vi "Initialize Session.vi"(7 "Acquisition Parameters In":T1={"Magnet Angle [deg]"=0.0, "Magnet Angles [deg]"=[], "DeltaVpp [v]"=0.0, "SEM [v]"=0.0, "DeltaVpp Thresh [v]"=0.0, "SEM Thresh [v]"=0.0, "Adaptive Processing"=FALSE, "Acquire Q"=FALSE, "Acquire Photos"=FALSE, "Adaptive Tuning"=FALSE, "Automated Matching"=FALSE, "X-Gradient [G/mm]"=0.0, "Y-Gradient [G/mm]"=0.0, "Z-Gradient [G/mm]"=0.0, "Central Field [G]"=0.0, "Scan Width [G]"=0.0, "Mod. Amp. [G]"=0.0, "Scan Time [s]"=0.0, "Pre-Scan Delay [ms]"=0, "Measurement Timeout [s]"=0.0, "Electromagnet Main Field [G]"=0.0, "Locked Central Field [G]"=0.0, "Scans Excluded"=0, "Scans Completed"=0, "No. Scans/Set"=0, "No. Scans for SNR"=0, "Field Locked Frequency [GHz]"=0.0, "Auto Set-based Field Center"=FALSE, "Prompt for oxy acquisition updates"=FALSE, "Oxy QA Scan?"=FALSE, "Exclude Bad Data"=FALSE, "Optimizing RF Power"=FALSE, "Gradients on/off"=TRUE, "Running Script"=FALSE, "Opto-Coupler Current [A]"=0.0, "Continuous Sweeping"=FALSE, "Sweep Rise Time [sec]"=0, "Reverse Sweep Central Field [G]"=0.0, "Forward Sweep Central Field [G]"=0.0, "Sweep Calibrated"=FALSE, "Modulation Calibrated"=FALSE, "First CheckCal Scan?"=FALSE, "AFC Field Correction"=FALSE, "OxyQAInit Scan Width [G]"=0.0, "OxyQAInit Mod. Amp. [G]"=0.0, "Scans Completed/Session"=0, "Acquire SpO2"=FALSE, "Acquire Temperature"=FALSE, "Over Mod"=FALSE} {"OxyQAInit Mod. Amp. [G]" min=0.0; "OxyQAInit Scan Width [G]" min=0.0; "Mod. Amp. [G]" min=0.0; "Scan Width [G]" min=0.0; "Measurement Timeout [s]" min=0.0; "Scan Time [s]" min=0.0; "Z-Gradient [G/mm]" min=0.0; "Y-Gradient [G/mm]" min=0.0; "X-Gradient [G/mm]" min=0.0; "SEM Thresh [v]" min=0.0; "DeltaVpp Thresh [v]" min=0.0; "SEM [v]" min=0.0}, 9 "Spectral Data In":T3={"PDT Amp [v]"=0.0, "RIS Amp [v]"=0.0, "B-Field"=[], "All In-Phase Scan Spectra"=[], "Model Select"=enum."OneCompRISTwoPDT", "Fit Each Scan"=FALSE, "PDT Center [g]"=0.0, "In-Phase Average Spectra"=[], "In-Phase Median Spectra"=[], "Out-Phase Median Spectra"=[], "Out-Phase Average Spectra"=[], "Fit Spectra"=[], "Fit No-Baseline Spectra"=[], "All Out-Phase Scan Spectra"=[], "Baseline Offset Correction"=FALSE, "In-Phase Offset [v]"=0.0, "Out-Phase Offset [v]"=0.0, "Ch2 Input\n(Balance)"=[], "Ch3 Input\n(Phase)"=[], "Ch4 Input\n(AFC)"=[], "Fit Pars"=[], "Fit Pars Errors"=[], "Fit Pars Labels"=[], "Raw Scan DAQ Data"=[], "Bad Scans Indicies"=[], "Good In-Phase Scan Spectra"=[], "Good Out-Phase Scan Spectra"=[], "Bad In-Phase Scan Spectra"=[], "Bad Out-Phase Scan Spectra"=[], "Number of bad scans"=0, "Fit History"=[], "PDT Amp. History/Set [v]"=[], "RIS Amp. History/Set [v]"=[], "RIS Amp. History/Scan [v]"=[], "All Shifted B-Fields"=[], "Good Shifted B-Fields"=[], "Ch5 Input\n(SpO2)"=[], "Ch6 Input\n(BPM)"=[], "Global SNR"=0.0, "Fit Error History"=[], "SNR History"=[]} {"Global SNR" min=0.0; "PDT Center [g]" min=0.0; "RIS Amp [v]" min=0.0; "PDT Amp [v]" min=0.0}, 10 "Measurement Information In":T7={"Comments"="", "Directory Input"="", "Data file path"=path "C:/Data/EPR Data", "Scripting File"=path "C:/Data/Configuration Script.csv", "Save Data"=FALSE, "Tooth size (d11) [mm]"=0.0, "Tooth size (d12) [mm]"=0.0, "Tooth size (d21) [mm]"=0.0, "Tooth size (d22) [mm]"=0.0, "Dose of Tooth [Gy]"=0.0, "Safe Shutdown?"=FALSE, "Gases Available"=[], "Database Username"="", "Database Password"="", "Database Login URL"="", "Database Upload URL"="", "Database Success URL"="", "Database XML URL"="", "Database Resonator URL"="", "Session Number"=0, "Set #"=0, "Resonator Operator"="", "Session Type"="", "Tooth/Sample ID"="", "Volunteer ID"="", "Computer Operator"="", "Volunteer Type"="", "Site/Tooth Selection (T8,T9)"="", "Resonator"="", "Measurement Site"="", "Non-standard session?"=FALSE, "EPR DAQ Version"="", "Session Path"=path "C:/Data/EPR Data", "Chosen Applied State"="", "Chosen Initial State"="", "Time of Transition"="", "DAQ Mode"=enum."Engineering", "pO2/Scan [mmHg]"=[], "pO2/Set [mmHg]"=[], "Linewidth (HWHM)/Scan [Gauss]"=[], "Linewidth (HWHM)/Set [Gauss]"=[], "pO2 Conversion"="", "Dose Calibration Cluster"={"Dose Response"={"grand_mean"=0.0292016, "slope"=0.0188720543}, "Dose Correction"={"Sex"=1, "a0"=7.719669421, "a1"=-2.746550736, "a2"=-0.186490355, "a3"=0.041922063, "a4"=-0.849147359, "a5"=0.14330063, "a6"=0.019930219, "A_n"=40.0, "H_n"=10.12, "Dose Correction"=FALSE}, "Dose Reporting"={"Reporting is"=TRUE, "sd_threshold [AU]"=0.06, "sd_model [Gy]"=0.66, "dosimetric_threshold [Gy]"=2.0, "Add intrasession errors is"=FALSE, "Prior Radiation?"=FALSE}}, "OxyChip Slope"=0.0, "OxyChip Intercept"=0.0, "QA Mode"=enum."Select QA Mode", "QA Session?"=FALSE, "Sample Type"=enum."Empty Resonator", "Report pO2/Scan"=FALSE, "Skip End Session Save"=FALSE, "Number of sites"=enum."# Probes", "Recipient Name"="", "Sender Name"="", "Recipient Email"="", "Transition State History"=[], "pO2 Report Times"=[], "Temperature [C]"=0.0, "+Error pO2/Scan [mmHg]"=[], "-Error pO2/Scan [mmHg]"=[], "+Error pO2/Set [mmHg]"=[], "-Error pO2/Set [mmHg]"=[], "Oxy Phase Exclusion Tolerance [rad]"=0.0, "Oxy Center Exclusion Tolerance [%]"=0.0, "Oxy Exclude Unacceptable"=FALSE, "Oxy Unacceptable Estimate Flags"=[], "Save Session PPT"=FALSE, "Flagged Bad Sets"=[]} {"Oxy Center Exclusion Tolerance [%]" format="%#_9g"; "Oxy Phase Exclusion Tolerance [rad]" format="%#_9g"; "Temperature [C]" format="%#_9g"; "OxyChip Intercept" format="%#_9g"; "OxyChip Slope" format="%#_9g"; "Dose Calibration Cluster"."Dose Reporting"."dosimetric_threshold [Gy]" format="%#_9g"; "Dose Calibration Cluster"."Dose Reporting"."sd_model [Gy]" format="%#_9g"; "Dose Calibration Cluster"."Dose Reporting"."sd_threshold [AU]" format="%#_9g"; "Dose Calibration Cluster"."Dose Correction"."H_n" format="%#_9g"; "Dose Calibration Cluster"."Dose Correction"."A_n" format="%#_9g"; "Dose Calibration Cluster"."Dose Correction"."a6" format="%#.9g"; "Dose Calibration Cluster"."Dose Correction"."a5" format="%#.9g"; "Dose Calibration Cluster"."Dose Correction"."a4" format="%#.9g"; "Dose Calibration Cluster"."Dose Correction"."a3" format="%#.9g"; "Dose Calibration Cluster"."Dose Correction"."a2" format="%#.9g"; "Dose Calibration Cluster"."Dose Correction"."a1" format="%#.9g"; "Dose Calibration Cluster"."Dose Correction"."a0" format="%#.9g"; "Dose Calibration Cluster"."Dose Correction"."Sex" items=["Male"=1, "Female"=0]; "Dose Calibration Cluster"."Dose Response"."slope" format="%#_9g"; "Dose Calibration Cluster"."Dose Response"."grand_mean" format="%#_9g"}, 11 "Hardware Parameters In":T2={"Scan Calibration [G/V]"=0.0, "Modulation Calibration [G/V]"=0.0, "Modulation Phase [deg]"=0.0, "Modulation Frequency [Hz]"=0.0, "Attenuation [dB]"=0, "Input Channel Count"=0, "Time constant"=7, "Sensitivity"=17, "Frequency Output Voltage [V]"=0.0, "Phase Output Voltage [V]"=0.0, "Lock-in Offset Compensation"=FALSE, "RF [GHz]"=0.0, "Q Start"=0.0, "Q End"=0.0, "Balance"=0.0, "Phase Error"=0.0, "AFC Error"=0.0, "AFC"=FALSE, "Magnet Rotation"=FALSE, "Balance Scaling Factor"=1.0, "Phase Error Scaling Factor"=1.0, "AFC Error Scaling Factor"=1.0, "Frequency Counter ID"="", "Sweep Waveform"=enum."Sawtooth", "Q-Factor Scale"=0.0, " Q-Data Scale"=0.0, " Q-Data Offset"=0.0, "Magnet Rotation Slope"=0.0, "Magnet Rotation Offset"=0.0, "Phase Sweep Resolution"=0.0, "Hardware Version Number"="", "Spectrometer ID Number"=0, "Spectrometer Name"="", "Lock in Saturation"=0.0, "Balance Threshold"=0.0, "Phase Error Threshold"=0.0, "AFC Error Threshold"=0.0, "Linear Actuator Length"=0.0, "Lock-in OK?"=FALSE, "Ignore Lock-in Comm. Failure"=FALSE, "Gradient Addresses"=[], "Gradient Calibrations [G/A*mm]"=[], "Gradient Power Supplies"=[], "Lock-in Address"="", "Magnet Type"=enum."RRI", "Camera Names"=[], "Sweep Limit [Gauss]"=0.0, "Modulation Limit [Gauss]"=0.0, "Balance Threshold Exceeded?"=FALSE, "Phase Threshold Exceeded?"=FALSE, "AFC Threshold Exceeded?"=FALSE, "Consecutive Re-tune attempts"=0, "Reverse Sweep Slope [sec]"=0.0, "Reverse Sweep Offset [G]"=0.0, "AFC Field Correction [V/MHz]"=0.0, "Active Gradients (X Y Z)"=[], "SpO2 Calibration [SpO2/V]"=1.0, "Heart Rate Calibration [BPM/V]"=1.0, "Thermocouple Channel"=""} {"Sensitivity" items=["", "2 nV", "5 nV", "10 nV", "20 nV", "50 nV", "100 nV", "200 nV", "500 nV", "1 uV", "2 uV", "5 uV", "10 uV", "20 uV", "50 uV", "100 uV", "200 uV", "500 uV", "1 mV", "2 mV", "5 mV", "10 mV", "20 mV", "50 mV", "100 mV", "200 mV", "500 mV", "1 V"]; "Time constant" items=["10 us", "20 us", "40 us", "80 us", "160 us", "320 us", "640 us", "5 ms", "10 ms", "20 ms", "50 ms", "100 ms", "200 ms", "500 ms", "1 s", "2 s", "5 s", "10 s", "20 s", "50 s", "100 s", "200 s", "500 s", "1 ks", "2 ks", "5 ks", "10 ks", "20 ks", "50 ks", "100 ks"]}) -> (0 "QSM Response":cluster{"Enum":T5, "Data":variant}[](array[cluster]), 1 "Spectral Data Out":T3={"PDT Amp [v]"=0.0, "RIS Amp [v]"=0.0, "B-Field"=[], "All In-Phase Scan Spectra"=[], "Model Select"=enum."OneCompRISTwoPDT", "Fit Each Scan"=FALSE, "PDT Center [g]"=0.0, "In-Phase Average Spectra"=[], "In-Phase Median Spectra"=[], "Out-Phase Median Spectra"=[], "Out-Phase Average Spectra"=[], "Fit Spectra"=[], "Fit No-Baseline Spectra"=[], "All Out-Phase Scan Spectra"=[], "Baseline Offset Correction"=FALSE, "In-Phase Offset [v]"=0.0, "Out-Phase Offset [v]"=0.0, "Ch2 Input\n(Balance)"=[], "Ch3 Input\n(Phase)"=[], "Ch4 Input\n(AFC)"=[], "Fit Pars"=[], "Fit Pars Errors"=[], "Fit Pars Labels"=[], "Raw Scan DAQ Data"=[], "Bad Scans Indicies"=[], "Good In-Phase Scan Spectra"=[], "Good Out-Phase Scan Spectra"=[], "Bad In-Phase Scan Spectra"=[], "Bad Out-Phase Scan Spectra"=[], "Number of bad scans"=0, "Fit History"=[], "PDT Amp. History/Set [v]"=[], "RIS Amp. History/Set [v]"=[], "RIS Amp. History/Scan [v]"=[], "All Shifted B-Fields"=[], "Good Shifted B-Fields"=[], "Ch5 Input\n(SpO2)"=[], "Ch6 Input\n(BPM)"=[], "Global SNR"=0.0, "Fit Error History"=[], "SNR History"=[]} {"Global SNR" min=0.0; "PDT Center [g]" min=0.0; "RIS Amp [v]" min=0.0; "PDT Amp [v]" min=0.0}, 2 "Measurement Information Out":T7={"Comments"="", "Directory Input"="", "Data file path"=path "C:/Data/EPR Data", "Scripting File"=path "C:/Data/Configuration Script.csv", "Save Data"=FALSE, "Tooth size (d11) [mm]"=0.0, "Tooth size (d12) [mm]"=0.0, "Tooth size (d21) [mm]"=0.0, "Tooth size (d22) [mm]"=0.0, "Dose of Tooth [Gy]"=0.0, "Safe Shutdown?"=FALSE, "Gases Available"=[], "Database Username"="", "Database Password"="", "Database Login URL"="", "Database Upload URL"="", "Database Success URL"="", "Database XML URL"="", "Database Resonator URL"="", "Session Number"=0, "Set #"=0, "Resonator Operator"="", "Session Type"="", "Tooth/Sample ID"="", "Volunteer ID"="", "Computer Operator"="", "Volunteer Type"="", "Site/Tooth Selection (T8,T9)"="", "Resonator"="", "Measurement Site"="", "Non-standard session?"=FALSE, "EPR DAQ Version"="", "Session Path"=path "C:/Data/EPR Data", "Chosen Applied State"="", "Chosen Initial State"="", "Time of Transition"="", "DAQ Mode"=enum."Engineering", "pO2/Scan [mmHg]"=[], "pO2/Set [mmHg]"=[], "Linewidth (HWHM)/Scan [Gauss]"=[], "Linewidth (HWHM)/Set [Gauss]"=[], "pO2 Conversion"="", "Dose Calibration Cluster"={"Dose Response"={"grand_mean"=0.0292016, "slope"=0.0188720543}, "Dose Correction"={"Sex"=1, "a0"=7.719669421, "a1"=-2.746550736, "a2"=-0.186490355, "a3"=0.041922063, "a4"=-0.849147359, "a5"=0.14330063, "a6"=0.019930219, "A_n"=40.0, "H_n"=10.12, "Dose Correction"=FALSE}, "Dose Reporting"={"Reporting is"=TRUE, "sd_threshold [AU]"=0.06, "sd_model [Gy]"=0.66, "dosimetric_threshold [Gy]"=2.0, "Add intrasession errors is"=FALSE, "Prior Radiation?"=FALSE}}, "OxyChip Slope"=0.0, "OxyChip Intercept"=0.0, "QA Mode"=enum."Select QA Mode", "QA Session?"=FALSE, "Sample Type"=enum."Empty Resonator", "Report pO2/Scan"=FALSE, "Skip End Session Save"=FALSE, "Number of sites"=enum."# Probes", "Recipient Name"="", "Sender Name"="", "Recipient Email"="", "Transition State History"=[], "pO2 Report Times"=[], "Temperature [C]"=0.0, "+Error pO2/Scan [mmHg]"=[], "-Error pO2/Scan [mmHg]"=[], "+Error pO2/Set [mmHg]"=[], "-Error pO2/Set [mmHg]"=[], "Oxy Phase Exclusion Tolerance [rad]"=0.0, "Oxy Center Exclusion Tolerance [%]"=0.0, "Oxy Exclude Unacceptable"=FALSE, "Oxy Unacceptable Estimate Flags"=[], "Save Session PPT"=FALSE, "Flagged Bad Sets"=[]} {"Oxy Center Exclusion Tolerance [%]" format="%#_9g"; "Oxy Phase Exclusion Tolerance [rad]" format="%#_9g"; "Temperature [C]" format="%#_9g"; "OxyChip Intercept" format="%#_9g"; "OxyChip Slope" format="%#_9g"; "Dose Calibration Cluster"."Dose Reporting"."dosimetric_threshold [Gy]" format="%#_9g"; "Dose Calibration Cluster"."Dose Reporting"."sd_model [Gy]" format="%#_9g"; "Dose Calibration Cluster"."Dose Reporting"."sd_threshold [AU]" format="%#_9g"; "Dose Calibration Cluster"."Dose Correction"."H_n" format="%#_9g"; "Dose Calibration Cluster"."Dose Correction"."A_n" format="%#_9g"; "Dose Calibration Cluster"."Dose Correction"."a6" format="%#.9g"; "Dose Calibration Cluster"."Dose Correction"."a5" format="%#.9g"; "Dose Calibration Cluster"."Dose Correction"."a4" format="%#.9g"; "Dose Calibration Cluster"."Dose Correction"."a3" format="%#.9g"; "Dose Calibration Cluster"."Dose Correction"."a2" format="%#.9g"; "Dose Calibration Cluster"."Dose Correction"."a1" format="%#.9g"; "Dose Calibration Cluster"."Dose Correction"."a0" format="%#.9g"; "Dose Calibration Cluster"."Dose Correction"."Sex" items=["Male"=1, "Female"=0]; "Dose Calibration Cluster"."Dose Response"."slope" format="%#_9g"; "Dose Calibration Cluster"."Dose Response"."grand_mean" format="%#_9g"}, 3 "Hardware Parameters Out":T2={"Scan Calibration [G/V]"=0.0, "Modulation Calibration [G/V]"=0.0, "Modulation Phase [deg]"=0.0, "Modulation Frequency [Hz]"=0.0, "Attenuation [dB]"=0, "Input Channel Count"=0, "Time constant"=7, "Sensitivity"=17, "Frequency Output Voltage [V]"=0.0, "Phase Output Voltage [V]"=0.0, "Lock-in Offset Compensation"=FALSE, "RF [GHz]"=0.0, "Q Start"=0.0, "Q End"=0.0, "Balance"=0.0, "Phase Error"=0.0, "AFC Error"=0.0, "AFC"=FALSE, "Magnet Rotation"=FALSE, "Balance Scaling Factor"=1.0, "Phase Error Scaling Factor"=1.0, "AFC Error Scaling Factor"=1.0, "Frequency Counter ID"="", "Sweep Waveform"=enum."Sawtooth", "Q-Factor Scale"=0.0, " Q-Data Scale"=0.0, " Q-Data Offset"=0.0, "Magnet Rotation Slope"=0.0, "Magnet Rotation Offset"=0.0, "Phase Sweep Resolution"=0.0, "Hardware Version Number"="", "Spectrometer ID Number"=0, "Spectrometer Name"="", "Lock in Saturation"=0.0, "Balance Threshold"=0.0, "Phase Error Threshold"=0.0, "AFC Error Threshold"=0.0, "Linear Actuator Length"=0.0, "Lock-in OK?"=FALSE, "Ignore Lock-in Comm. Failure"=FALSE, "Gradient Addresses"=[], "Gradient Calibrations [G/A*mm]"=[], "Gradient Power Supplies"=[], "Lock-in Address"="", "Magnet Type"=enum."RRI", "Camera Names"=[], "Sweep Limit [Gauss]"=0.0, "Modulation Limit [Gauss]"=0.0, "Balance Threshold Exceeded?"=FALSE, "Phase Threshold Exceeded?"=FALSE, "AFC Threshold Exceeded?"=FALSE, "Consecutive Re-tune attempts"=0, "Reverse Sweep Slope [sec]"=0.0, "Reverse Sweep Offset [G]"=0.0, "AFC Field Correction [V/MHz]"=0.0, "Active Gradients (X Y Z)"=[], "SpO2 Calibration [SpO2/V]"=1.0, "Heart Rate Calibration [BPM/V]"=1.0, "Thermocouple Channel"=""} {"Sensitivity" items=["", "2 nV", "5 nV", "10 nV", "20 nV", "50 nV", "100 nV", "200 nV", "500 nV", "1 uV", "2 uV", "5 uV", "10 uV", "20 uV", "50 uV", "100 uV", "200 uV", "500 uV", "1 mV", "2 mV", "5 mV", "10 mV", "20 mV", "50 mV", "100 mV", "200 mV", "500 mV", "1 V"]; "Time constant" items=["10 us", "20 us", "40 us", "80 us", "160 us", "320 us", "640 us", "5 ms", "10 ms", "20 ms", "50 ms", "100 ms", "200 ms", "500 ms", "1 s", "2 s", "5 s", "10 s", "20 s", "50 s", "100 s", "200 s", "500 s", "1 ks", "2 ks", "5 ks", "10 ks", "20 ks", "50 ks", "100 ks"]}, 4 "error out":errorcluster, 5 "Acquisition Parameters Out":T1={"Magnet Angle [deg]"=0.0, "Magnet Angles [deg]"=[], "DeltaVpp [v]"=0.0, "SEM [v]"=0.0, "DeltaVpp Thresh [v]"=0.0, "SEM Thresh [v]"=0.0, "Adaptive Processing"=FALSE, "Acquire Q"=FALSE, "Acquire Photos"=FALSE, "Adaptive Tuning"=FALSE, "Automated Matching"=FALSE, "X-Gradient [G/mm]"=0.0, "Y-Gradient [G/mm]"=0.0, "Z-Gradient [G/mm]"=0.0, "Central Field [G]"=0.0, "Scan Width [G]"=0.0, "Mod. Amp. [G]"=0.0, "Scan Time [s]"=0.0, "Pre-Scan Delay [ms]"=0, "Measurement Timeout [s]"=0.0, "Electromagnet Main Field [G]"=0.0, "Locked Central Field [G]"=0.0, "Scans Excluded"=0, "Scans Completed"=0, "No. Scans/Set"=0, "No. Scans for SNR"=0, "Field Locked Frequency [GHz]"=0.0, "Auto Set-based Field Center"=FALSE, "Prompt for oxy acquisition updates"=FALSE, "Oxy QA Scan?"=FALSE, "Exclude Bad Data"=FALSE, "Optimizing RF Power"=FALSE, "Gradients on/off"=TRUE, "Running Script"=FALSE, "Opto-Coupler Current [A]"=0.0, "Continuous Sweeping"=FALSE, "Sweep Rise Time [sec]"=0, "Reverse Sweep Central Field [G]"=0.0, "Forward Sweep Central Field [G]"=0.0, "Sweep Calibrated"=FALSE, "Modulation Calibrated"=FALSE, "First CheckCal Scan?"=FALSE, "AFC Field Correction"=FALSE, "OxyQAInit Scan Width [G]"=0.0, "OxyQAInit Mod. Amp. [G]"=0.0, "Scans Completed/Session"=0, "Acquire SpO2"=FALSE, "Acquire Temperature"=FALSE, "Over Mod"=FALSE} {"OxyQAInit Mod. Amp. [G]" min=0.0; "OxyQAInit Scan Width [G]" min=0.0; "Mod. Amp. [G]" min=0.0; "Scan Width [G]" min=0.0; "Measurement Timeout [s]" min=0.0; "Scan Time [s]" min=0.0; "Z-Gradient [G/mm]" min=0.0; "Y-Gradient [G/mm]" min=0.0; "X-Gradient [G/mm]" min=0.0; "SEM Thresh [v]" min=0.0; "DeltaVpp Thresh [v]" min=0.0; "SEM [v]" min=0.0})   [LabVIEW 2016]
uses:
  Types/Measurement Information.ctl
  Analysis/Dose Calculation and Reporting/Dose Calculation Control.ctl
  Types/Sample Type.ctl
  Types/State Control.ctl
  Types/Spectral Data.ctl
  Types/Fitting Model Selection.ctl
  Types/Hardware Parameters.ctl
  Types/Acquisition Parameters.ctl
  Types/Global Variables.vi
panel:
  in  "Number of sites":enum16{"# Probes", "1", "2", "3", "4"}(ring) caption="Number of Probes\n(only used for IR)"
  in  "QA Mode":T6(ring)
  in  "Check Box for Nonstandard Use":bool
  in  "Session Type":u16(ring)=1 items=["QA", "VITRO", "VIVO"]
  in  "Computer\nOperator(initials)":string
  in  "Resonator \nOperator(initials)":string
  in  "stop":bool
  # "Session Parameters"
  # "Gradients"
  # "Field"
  # "Scans and Sets"
  # "Timing"
  # "Adaptive Dosimetric \nData Processing"
  # "Gradients"
  # "Field"
  # "Scans and Sets"
  # "Timing"
  # "Adaptive Dosimetric \nData Processing"
  # "Bridge I/O"
  # "Magnet Rotation"
  # "Field Calibration"
  # "Lock In Amplifier"
  # "Spectrometer Information"
  # "DAQ Settings"
  # "Gradient Coils and Field"
  # "X"
  # "Y"
  # "Z"
  # "Q-Measurements"
  # "Bridge I/O"
  # "Magnet Rotation"
  # "Field Calibration"
  # "Lock In Amplifier"
  # "Spectrometer Information"
  # "DAQ Settings"
  # "Gradient Coils and Field"
  # "X"
  # "Y"
  # "Z"
  # "Q-Measurements"
  # "Session Information"
  # "Oximetric Data and Information"
  # "Email"
  # "Tooth Information"
  # "Database"
  # "Session Information"
  # "Oximetric Data and Information"
  # "Email"
  # "Tooth Information"
  # "Database"
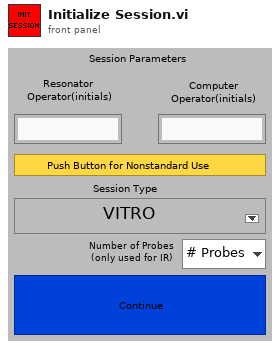
[diagram p1: front panel]
types:
  T1 = typedef "Acquisition Parameters.ctl" = cluster{"Magnet Angle [deg]":dbl, "Magnet Angles [deg]":dbl[], "DeltaVpp [v]":dbl, "SEM [v]":dbl, "DeltaVpp Thresh [v]":dbl, "SEM Thresh [v]":dbl, "Adaptive Processing":bool, "Acquire Q":bool, "Acquire Photos":bool, "Adaptive Tuning":bool, "Automated Matching":bool, "X-Gradient [G/mm]":dbl, "Y-Gradient [G/mm]":dbl, "Z-Gradient [G/mm]":dbl, "Central Field [G]":dbl, "Scan Width [G]":dbl, "Mod. Amp. [G]":dbl, "Scan Time [s]":dbl, "Pre-Scan Delay [ms]":u32, "Measurement Timeout [s]":dbl, "Electromagnet Main Field [G]":dbl, "Locked Central Field [G]":dbl, "Scans Excluded":u32, "Scans Completed":u32, "No. Scans/Set":u32, "No. Scans for SNR":u32, "Field Locked Frequency [GHz]":dbl, "Auto Set-based Field Center":bool, "Prompt for oxy acquisition updates":bool, "Oxy QA Scan?":bool, "Exclude Bad Data":bool, "Optimizing RF Power":bool, "Gradients on/off":bool, "Running Script":bool, "Opto-Coupler Current [A]":dbl, "Continuous Sweeping":bool, "Sweep Rise Time [sec]":u32, "Reverse Sweep Central Field [G]":dbl, "Forward Sweep Central Field [G]":dbl, "Sweep Calibrated":bool, "Modulation Calibrated":bool, "First CheckCal Scan?":bool, "AFC Field Correction":bool, "OxyQAInit Scan Width [G]":dbl, "OxyQAInit Mod. Amp. [G]":dbl, "Scans Completed/Session":u32, "Acquire SpO2":bool, "Acquire Temperature":bool, "Over Mod":bool}
  T2 = typedef "Hardware Parameters.ctl" = cluster{"Scan Calibration [G/V]":dbl, "Modulation Calibration [G/V]":dbl, "Modulation Phase [deg]":dbl, "Modulation Frequency [Hz]":dbl, "Attenuation [dB]":u16, "Input Channel Count":i32, "Time constant":u16, "Sensitivity":u16, "Frequency Output Voltage [V]":dbl, "Phase Output Voltage [V]":dbl, "Lock-in Offset Compensation":bool, "RF [GHz]":dbl, "Q Start":dbl, "Q End":dbl, "Balance":dbl, "Phase Error":dbl, "AFC Error":dbl, "AFC":bool, "Magnet Rotation":bool, "Balance Scaling Factor":dbl, "Phase Error Scaling Factor":dbl, "AFC Error Scaling Factor":dbl, "Frequency Counter ID":string, "Sweep Waveform":enum16{"Sine Wave", "Square Wave", "Sawtooth", "Triangle Wave"}, "Q-Factor Scale":dbl, " Q-Data Scale":dbl, " Q-Data Offset":dbl, "Magnet Rotation Slope":dbl, "Magnet Rotation Offset":dbl, "Phase Sweep Resolution":dbl, "Hardware Version Number":string, "Spectrometer ID Number":i32, "Spectrometer Name":string, "Lock in Saturation":dbl, "Balance Threshold":dbl, "Phase Error Threshold":dbl, "AFC Error Threshold":dbl, "Linear Actuator Length":dbl, "Lock-in OK?":bool, "Ignore Lock-in Comm. Failure":bool, "Gradient Addresses":string[], "Gradient Calibrations [G/A*mm]":dbl[], "Gradient Power Supplies":string[], "Lock-in Address":refnum<visa-resource-name>, "Magnet Type":enum16{"RRI", "BARDA", "Whole Body Permanent", "RRI Electromagnet"}, "Camera Names":string[], "Sweep Limit [Gauss]":dbl, "Modulation Limit [Gauss]":dbl, "Balance Threshold Exceeded?":bool, "Phase Threshold Exceeded?":bool, "AFC Threshold Exceeded?":bool, "Consecutive Re-tune attempts":i32, "Reverse Sweep Slope [sec]":dbl, "Reverse Sweep Offset [G]":dbl, "AFC Field Correction [V/MHz]":dbl, "Active Gradients (X Y Z)":bool[], "SpO2 Calibration [SpO2/V]":dbl, "Heart Rate Calibration [BPM/V]":dbl, "Thermocouple Channel":tag}
  T3 = typedef "Spectral Data.ctl" = cluster{"PDT Amp [v]":dbl, "RIS Amp [v]":dbl, "B-Field":dbl[], "All In-Phase Scan Spectra":dbl[][], "Model Select":T4, "Fit Each Scan":bool, "PDT Center [g]":dbl, "In-Phase Average Spectra":dbl[], "In-Phase Median Spectra":dbl[], "Out-Phase Median Spectra":dbl[], "Out-Phase Average Spectra":dbl[], "Fit Spectra":dbl[], "Fit No-Baseline Spectra":dbl[], "All Out-Phase Scan Spectra":dbl[][], "Baseline Offset Correction":bool, "In-Phase Offset [v]":dbl, "Out-Phase Offset [v]":dbl, "Ch2 Input\n(Balance)":dbl[], "Ch3 Input\n(Phase)":dbl[], "Ch4 Input\n(AFC)":dbl[], "Fit Pars":dbl[], "Fit Pars Errors":dbl[], "Fit Pars Labels":string[], "Raw Scan DAQ Data":dbl[][], "Bad Scans Indicies":i32[], "Good In-Phase Scan Spectra":dbl[][], "Good Out-Phase Scan Spectra":dbl[][], "Bad In-Phase Scan Spectra":dbl[][], "Bad Out-Phase Scan Spectra":dbl[][], "Number of bad scans":i32, "Fit History":dbl[][], "PDT Amp. History/Set [v]":dbl[], "RIS Amp. History/Set [v]":dbl[], "RIS Amp. History/Scan [v]":dbl[], "All Shifted B-Fields":dbl[][], "Good Shifted B-Fields":dbl[][], "Ch5 Input\n(SpO2)":dbl[], "Ch6 Input\n(BPM)":dbl[], "Global SNR":dbl, "Fit Error History":dbl[][], "SNR History":dbl[]}
  T4 = typedef "Fitting Model Selection.ctl" = enum16{"OneCompRIS", "OneCompRISTwoPDT", "OneCompRISRev", "OneCompRISTwoPDTRev", "LiPc", "TwoLiPc", "ThreeLiPc", "FourLiPc", "PDTCalibration", "CE_Ink", "Printex", "MelaninTwoPDT"}
  T5 = typedef "State Control.ctl" = enum16{"Startup", "Read Config File", "Initilize Optional Hardware", "Idle", "New Session", "Read GUI Pars", "Configure Hardware", "Initialize Set", "Pre-Scan", "Scan", "Post-Scan", "Exit Set", "Automated Tuning", "Manual Tuning", "Check Calibration", "Optimize RF Power", "Test Scan", "Set Oxy QA-Scan Pars", "Find Peaks", "Update from Cursors", "Flag Bad Set", "Mark transition time", "Measure Q", "Measure Noise", "Rotate Magnet", "Lock Field", "Engineering Tuning", "Zero Voltages", "Update Center Field", "Refit Data", "Open Session Data Folder", "AfterSave", "Undo Auto Update Pars", "Read from Script", "End Session", "Quit Software", "Error"}
  T6 = enum16{"Select QA Mode", "QA-Start/End", "QA-Mid", "QA-Weekly", "QA-Eng", "Check Calibration"}
  T7 = typedef "Measurement Information.ctl" = cluster{"Comments":string, "Directory Input":string, "Data file path":path, "Scripting File":path, "Save Data":bool, "Tooth size (d11) [mm]":dbl, "Tooth size (d12) [mm]":dbl, "Tooth size (d21) [mm]":dbl, "Tooth size (d22) [mm]":dbl, "Dose of Tooth [Gy]":dbl, "Safe Shutdown?":bool, "Gases Available":string[], "Database Username":string, "Database Password":string, "Database Login URL":string, "Database Upload URL":string, "Database Success URL":string, "Database XML URL":string, "Database Resonator URL":string, "Session Number":i32, "Set #":u32, "Resonator Operator":string, "Session Type":string, "Tooth/Sample ID":string, "Volunteer ID":string, "Computer Operator":string, "Volunteer Type":string, "Site/Tooth Selection (T8,T9)":string, "Resonator":string, "Measurement Site":string, "Non-standard session?":bool, "EPR DAQ Version":string, "Session Path":path, "Chosen Applied State":string, "Chosen Initial State":string, "Time of Transition":string, "DAQ Mode":enum16{"Engineering", "Dosimetry", "Oximetry"}, "pO2/Scan [mmHg]":dbl[][], "pO2/Set [mmHg]":dbl[][], "Linewidth (HWHM)/Scan [Gauss]":dbl[][], "Linewidth (HWHM)/Set [Gauss]":dbl[][], "pO2 Conversion":string, "Dose Calibration Cluster":T8, "OxyChip Slope":dbl, "OxyChip Intercept":dbl, "QA Mode":enum16{"Select QA Mode", "QA-Start/End", "QA-Mid", "QA-Weekly", "QA-Eng", "Check Calibration"}, "QA Session?":bool, "Sample Type":T9, "Report pO2/Scan":bool, "Skip End Session Save":bool, "Number of sites":enum16{"# Probes", "1", "2", "3", "4"}, "Recipient Name":string, "Sender Name":string, "Recipient Email":string, "Transition State History":string[], "pO2 Report Times":string[], "Temperature [C]":dbl, "+Error pO2/Scan [mmHg]":dbl[][], "-Error pO2/Scan [mmHg]":dbl[][], "+Error pO2/Set [mmHg]":dbl[][], "-Error pO2/Set [mmHg]":dbl[][], "Oxy Phase Exclusion Tolerance [rad]":dbl, "Oxy Center Exclusion Tolerance [%]":dbl, "Oxy Exclude Unacceptable":bool, "Oxy Unacceptable Estimate Flags":bool[], "Save Session PPT":bool, "Flagged Bad Sets":u32[]}
  T8 = typedef "Dose Calculation Control.ctl" = cluster{"Dose Response":cluster{"grand_mean":dbl, "slope":dbl}, "Dose Correction":cluster{"Sex":u16, "a0":dbl, "a1":dbl, "a2":dbl, "a3":dbl, "a4":dbl, "a5":dbl, "a6":dbl, "A_n":dbl, "H_n":dbl, "Dose Correction":bool}, "Dose Reporting":cluster{"Reporting is":bool, "sd_threshold [AU]":dbl, "sd_model [Gy]":dbl, "dosimetric_threshold [Gy]":dbl, "Add intrasession errors is":bool, "Prior Radiation?":bool}}
  T9 = typedef "Sample Type.ctl" = enum16{"Empty Resonator", "IRS", "BallZero", "Irradiated Tooth", "Non-irradiated Tooth", "OxyChip", "LiPc", "PDT", "India Ink"}
  T10 = enum8{"Enabled", "Disabled", "Disabled and Grayed Out"}
  T11 = enum16{"Select QA Mode", "QA-Start/End", "QA-Mid", "QA-Eng"}[]
  T12 = enum16{"Select QA Mode", "QA-Start/End", "QA-Mid", "QA-Weekly", "QA-Eng", "Check Calibration"}[]
  T13 = cluster{"Resonator Data File":string[], "In Vivo Data File":string[], "Volunteer ID":string[], "Tooth Position File":string[], "Sample Selection":string[], "Tooth Data File":string[], "Ball Zero Options":string[], "Fraction of Oxygen":string[], "Gases Used":string[], "IRS Options":string[], "Standard File":string[], "Tooth Strings":string[]}
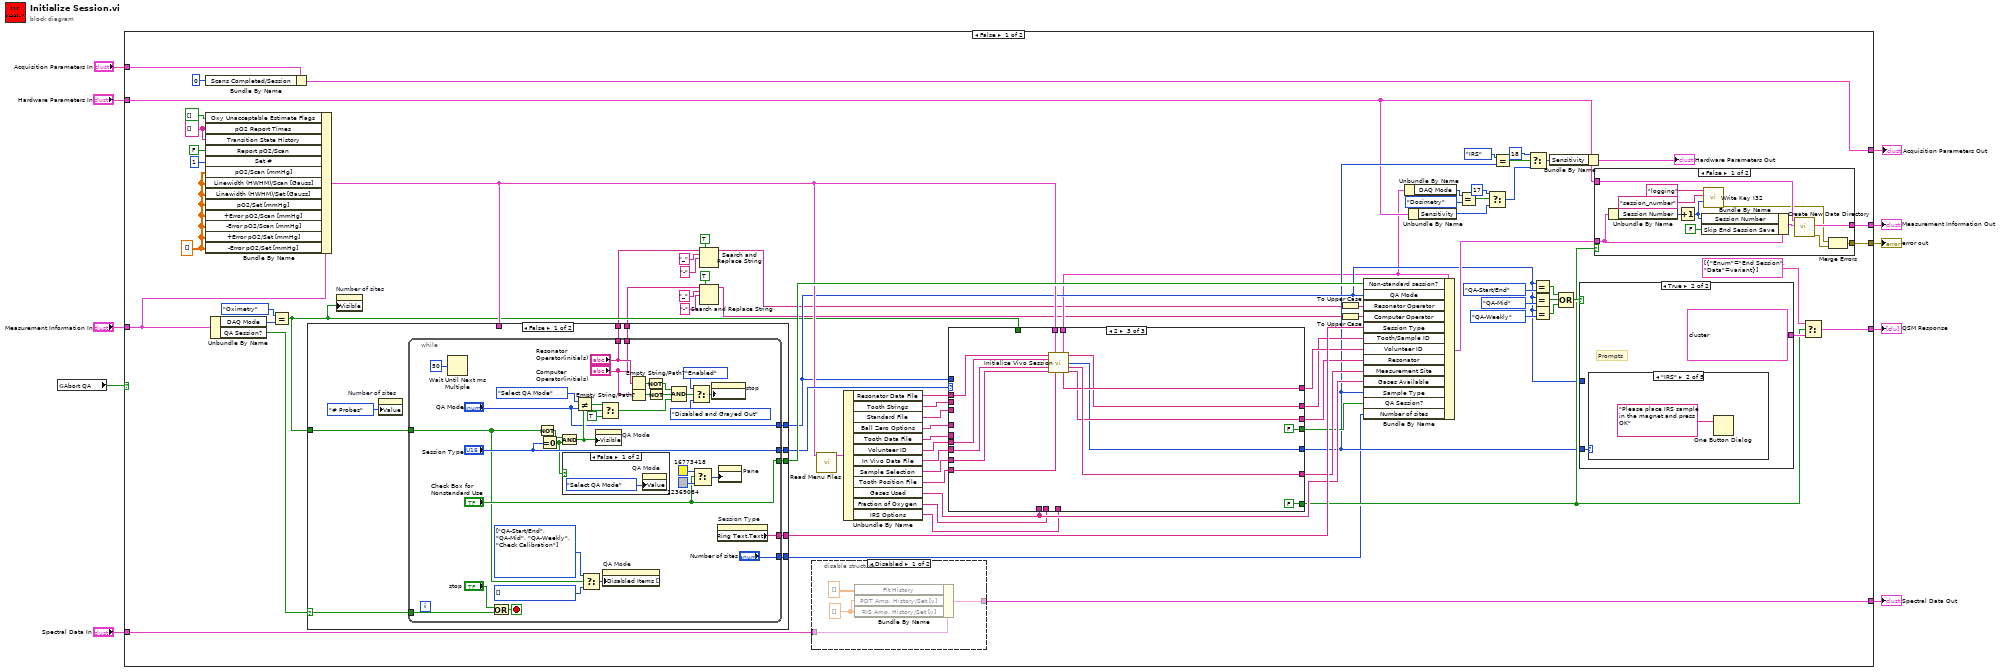
[diagram p0: block diagram]
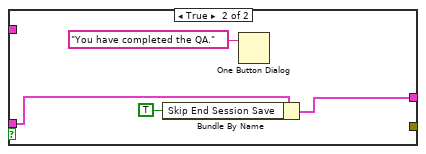
[diagram p3: hidden frame]
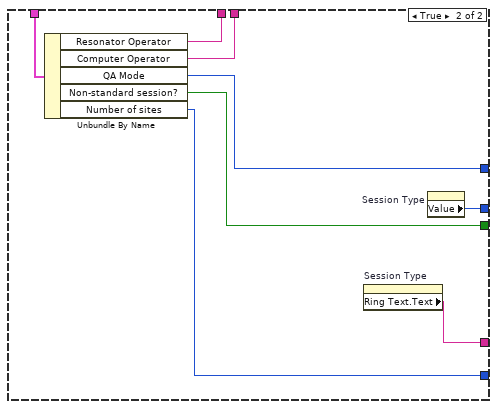
[diagram p5: hidden frame]
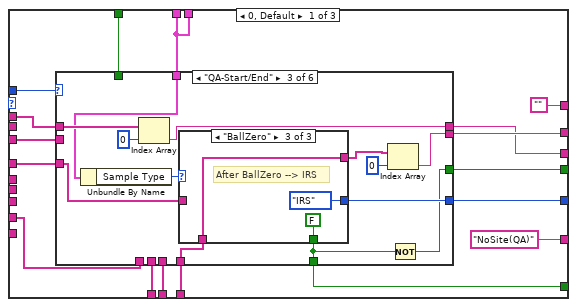
[diagram p6: hidden frame]
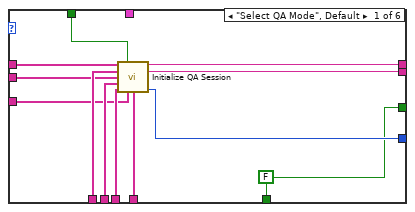
[diagram p7: hidden frame]
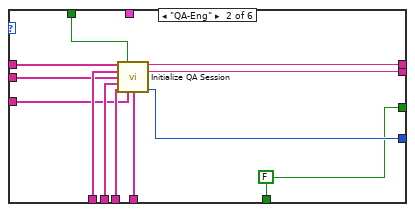
[diagram p8: hidden frame]
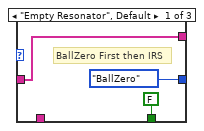
[diagram p9: hidden frame]
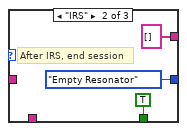
[diagram p10: hidden frame]
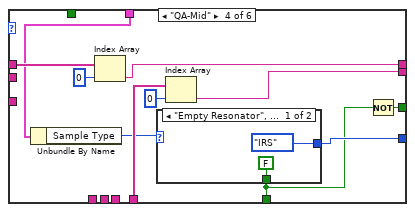
[diagram p11: hidden frame]
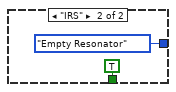
[diagram p12: hidden frame]
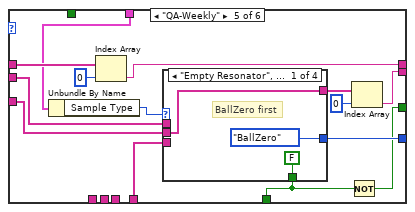
[diagram p13: hidden frame]
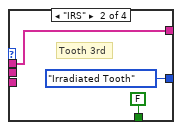
[diagram p14: hidden frame]
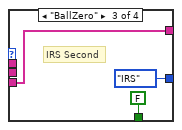
[diagram p15: hidden frame]
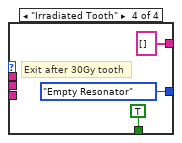
[diagram p16: hidden frame]
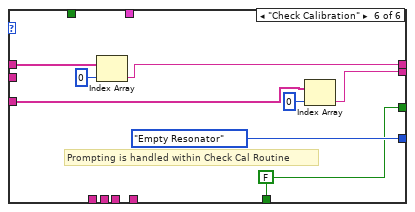
[diagram p17: hidden frame]
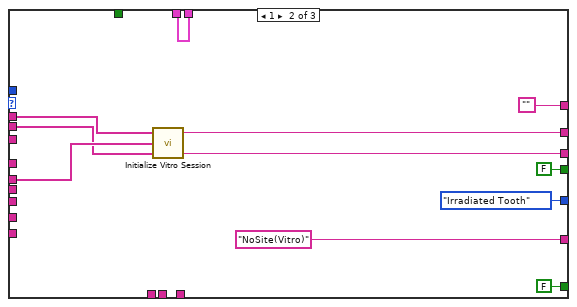
[diagram p18: hidden frame]
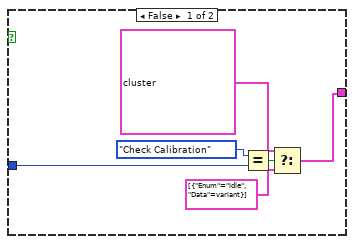
[diagram p19: hidden frame]
diagram:
  n1 = global read "Global Variables.vi" "Abort QA"() -> (w3:bool)
  n2 = case shown="False" w3 {
    tunnel: [w78 cluster{"Enum":T5, "Data":variant}[] [{"Enum"=enum."End Session", "Data"=variant}]] -> w10
    tunnel: "Spectral Data In" -> [w56 w313]
    tunnel: "Measurement Information In" -> [w55 w312]
    tunnel: [w53 w314] -> w7
    tunnel: [w47 w313] -> w6
    tunnel: [w46 errorcluster {"status"=FALSE, "code"=0, "source"=""} ("error IO")] -> w5
    tunnel: "Hardware Parameters In" -> [w39 _]
    tunnel: "Acquisition Parameters In" -> [w28 w311]
    tunnel: [w24 w311] -> w1
    frame False {
      w25 = string[] [] ("Transition State History")
      w23 = dbl[][] [] ("pO2/Scan [mmHg]")
      n3 = Bundle By Name(cluster=w28, "Scans Completed/Session"=u32 0) -> (w24:T1)
      n4 = Bundle By Name(cluster=w55, "Oxy Unacceptable Estimate Flags"=bool[] [], "pO2 Report Times"=w25, "Transition State History"=w25, "Report pO2/Scan"=FALSE, "Set #"=u32 1, "pO2/Scan [mmHg]"=w23, "Linewidth (HWHM)/Scan [Gauss]"=w23, "Linewidth (HWHM)/Set [Gauss]"=w23, "pO2/Set [mmHg]"=w23, "+Error pO2/Scan [mmHg]"=w23, "-Error pO2/Scan [mmHg]"=w23, "+Error pO2/Set [mmHg]"=w23, "-Error pO2/Set [mmHg]"=w23) -> (w50:T7)
      n5 = Unbundle By Name(w55) -> ("DAQ Mode"=w22:enum16{"Engineering", "Dosimetry", "Oximetry"}, "QA Session?"=w51:bool)
      n6 = Equal?(x=enum16{"Engineering", "Dosimetry", "Oximetry"}."Oximetry" ("DAQ Mode"), y=w22) -> (x = y?=w31:bool)
      n7 = case shown="False" w51 {
        selector: w51 -> [w114 _]
        tunnel: [w120 w162] -> w89
        tunnel: [w119 w156] -> w84
        tunnel: [w118 w160] -> w14
        tunnel: [w117 w159] -> w12
        tunnel: w31 -> [w113 _]
        tunnel: [w116 w157] -> w76
        tunnel: [w115 w158] -> w48
        tunnel: w50 -> [_ w161]
        tunnel: [w112 w155] -> w30
        frame False {
          n8 = property on="Number of sites" class="Enum (strict)"("Value"=enum16{"# Probes", "1", "2", "3", "4"}."# Probes" ("Number of sites")) -> ()  [unwired: 2 in, 2 out]
          n9 = while {
            tunnel: ["Session Type"] -> w116
            tunnel: ["Resonator \nOperator(initials)"] -> w118
            tunnel: ["Computer\nOperator(initials)"] -> w117
            tunnel: ["Check Box for Nonstandard Use"] -> w119
            tunnel: w113 -> [w126]
            tunnel: ["QA Mode"] -> w115
            tunnel: [w130] -> w120
            tunnel: w114 -> [w124]
            tunnel: ["Number of sites"] -> w112
            stop <- w123 stop-if-true
            w129 = T11 [] items=["Select QA Mode", "QA-Start/End", "QA-Mid", "QA-Eng"] ("Disabled Items []")
            w128 = T12 [enum."QA-Start/End", enum."QA-Mid", enum."QA-Weekly", enum."Check Calibration"] items=["Select QA Mode", "QA-Start/End", "QA-Mid", "QA-Weekly", "QA-Eng", "Check Calibration"] ("Disabled Items []")
            n10 = Wait Until Next ms Multiple(millisecond multiple=u32 50) -> ()  [unwired: 1 out]
            n11 = Or(x="stop", y=w124) -> (x .or. y?=w123:bool)
            n12 = Not(x=w126) -> (.not. x?=w137:bool)
            n13 = Equal To 0?(x="Session Type") -> (x = 0?=w122:bool)
            n14 = And(x=w137, y=w122) -> (x .and. y?=w135:bool)
            n15 = case shown="False" w122 {
              frame False {
                n16 = property on="QA Mode" class="Enum (strict)"("Value"=T6."Select QA Mode" ("QA Mode")) -> ()  [unwired: 2 in, 2 out]
              }
              frame True {
              }
            }
            n17 = Not Equal?(x=T6."Select QA Mode" ("QA Mode"), y="QA Mode") -> (x != y?=w134:bool)
            n18 = Select(t=w128, s=w126, f=w129) -> (s? t:f=w127:u16[])
            n19 = property on="QA Mode" class="Enum (strict)"("Visible"=w135) -> ()  [unwired: 2 in, 2 out]
            n20 = Select(t=w134, s=w135, f=TRUE) -> (s? t:f=w132:bool)
            n21 = property on="QA Mode" class="Enum (strict)"("Disabled Items []"=w127) -> ()  [unwired: 2 in, 2 out]
            n22 = Empty String/Path?(string/path="Resonator \nOperator(initials)") -> (empty?=w146:bool)
            n23 = Empty String/Path?(string/path="Computer\nOperator(initials)") -> (empty?=w145:bool)
            n24 = Not(x=w146) -> (.not. x?=w144:bool)
            n25 = Not(x=w145) -> (.not. x?=w143:bool)
            n26 = Compound Arithmetic op=AND(w144, w143, w132) -> (w142:bool)
            n27 = Select(t=T10."Enabled" ("Disabled"), s=w142, f=T10."Disabled and Grayed Out" ("Disabled")) -> (s? t:f=w139:T10)
            n28 = Select(t=u32 16773418, s="Check Box for Nonstandard Use", f=u32 12369084) -> (s? t:f=w152:u32)
            n29 = property on="stop" class="Bool"("DisabledEnum"=w139) -> ()  [unwired: 2 in, 2 out]
            n30 = property on="Session Type" class="Ring (strict)"() -> ("Ring Text.Text"=w130:string)  [unwired: 2 in, 2 out]
            n31 = property on="Pane" class="Pane"("PaneColor"=w152) -> ()  [unwired: 2 in, 2 out]
          }
        }
        frame True {
          n32 = Unbundle By Name(w161) -> ("Resonator Operator"=w160:string, "Computer Operator"=w159:string, "QA Mode"=w158:T6, "Non-standard session?"=w156:bool, "Number of sites"=w155:enum16{"# Probes", "1", "2", "3", "4"})
          n33 = property on="Session Type" class="Ring (strict)"() -> ("Ring Text.Text"=w162:string)  [unwired: 2 in, 2 out]
          n34 = property on="Session Type" class="Ring (strict)"() -> ("Value"=w157:u16)  [unwired: 2 in, 2 out]
        }
      }
      n35 = property on="Number of sites" class="Enum (strict)"("Visible"=w31) -> ()  [unwired: 2 in, 2 out]
      n36 = Search and Replace String(replace all?=TRUE ("replace all? (F)"), input string=w14, search string="_", replace string="-" ("replace string (\"\")")) -> (result string=w13:string)  [unwired: 4 in, 3 out]
      n37 = Search and Replace String(replace all?=TRUE ("replace all? (F)"), input string=w12, search string="_", replace string="-" ("replace string (\"\")")) -> (result string=w11:string)  [unwired: 4 in, 3 out]
      n38 = disable-structure shown="Disabled" {
        disable-tunnel: w56 -> [w92 w94]
        disable-tunnel: [w91 w94] -> w47
        frame Disabled {
          w90 = dbl[] [] ("PDT Amp. History/Set [v]")
          n39 = Bundle By Name(cluster=w92, "Fit History"=dbl[][] [], "PDT Amp. History/Set [v]"=w90, "RIS Amp. History/Set [v]"=w90) -> (w91:T3)
        }
        frame Enabled {
        }
      }
      n40 = call "Read Menu Files.vi"("Measurement Information In"=w50) -> ("Menu Selections Output"=w75:T13)  [unwired: 10 in]
      n41 = Unbundle By Name(w75) -> ("Resonator Data File"=w74:string[], "Tooth Strings"=w73:string[], "Standard File"=w72:string[], "Ball Zero Options"=w71:string[], "Tooth Data File"=w70:string[], "Volunteer ID"=w69:string[], "In Vivo Data File"=w68:string[], "Sample Selection"=w67:string[], "Tooth Position File"=w66:string[], "Gases Used"=w85:string[], "Fraction of Oxygen"=w65:string[], "IRS Options"=w64:string[])
      n42 = case shown="2" w76 {
        tunnel: w70 -> [_ w284 _]
        tunnel: w74 -> [w179 w285 w299]
        tunnel: w73 -> [_ w283 _]
        tunnel: w68 -> [_ _ w297]
        tunnel: w66 -> [_ _ w294]
        tunnel: w69 -> [_ _ w298]
        tunnel: w65 -> [w178 _ _]
        tunnel: w85 -> [w176 _ _]
        tunnel: w67 -> [w177 _ w296]
        tunnel: ["NoSite(QA)" ("Measurement Site") "NoSite(Vitro)" ("Measurement Site") w295] -> w86
        tunnel: ["" "" w293] -> w88
        tunnel: [w173 w280 w291] -> w81
        tunnel: [w172 w279 w292] -> w87
        tunnel: w31 -> [w171 _ _]
        tunnel: w50 -> [w165 w278 w290]
        tunnel: [w165 w278 w289] -> w32
        tunnel: w71 -> [w170 _ _]
        tunnel: w64 -> [w169 _ _]
        tunnel: w72 -> [w168 _ _]
        tunnel: w48 -> [w167 _ _]
        tunnel: [w166 Sample_Type."Irradiated Tooth" ("Sample Type") w287] -> w40
        tunnel: [w164 FALSE ("s") FALSE ("s")] -> w49
        tunnel: [w163 FALSE ("s") FALSE ("s")] -> w52
        frame 0, Default {
          n43 = case shown="\"QA-Start/End\"" w167 {
            tunnel: w179 -> [w191 w203 w216 w236 w254 w274]
            tunnel: w178 -> [w190 w202 _ _ _ _]
            tunnel: w177 -> [w189 w201 _ _ _ _]
            tunnel: w176 -> [w188 w200 _ _ _ _]
            tunnel: [w187 w199 w209 w231 w248 w269] -> w173
            tunnel: [w186 w198 w214 w235 w253 w273] -> w172
            tunnel: w171 -> [w185 w197 _ _ _ _]
            tunnel: w170 -> [w184 w196 w206 _ w250 w268]
            tunnel: w169 -> [w183 w195 w208 w232 w246 _]
            tunnel: w168 -> [w182 w194 _ _ w245 _]
            tunnel: [w181 w193 w211 w230 w251 Sample_Type."Empty Resonator" ("Sample Type")] -> w166
            tunnel: w165 -> [_ _ w213 w228 w243 _]
            tunnel: [w180 w192 w205 w227 w242 w267] -> w164
            tunnel: [w180 w192 w204 w226 w241 w267] -> w163
            frame "Select QA Mode", Default {
              w180 = FALSE ("s")
              n44 = call "Initialize QA Session.vi"("resonator labels"=w191, "Oximetry Mode?"=w185, "Sample Selection"=w189, "Standard Options"=w182, "Gases Used"=w188, "Fraction of Inhaled Oxygen"=w190, "BallZero Options"=w184, "IRS Options"=w183) -> ("Resonator ID"=w186:string, "Sample Selected"=w187:string, "Sample Type"=w181:T9)  [unwired: 4 in, 1 out]
            }
            frame "QA-Eng" {
              w192 = FALSE ("s")
              n45 = call "Initialize QA Session.vi"("resonator labels"=w203, "Oximetry Mode?"=w197, "Sample Selection"=w201, "Standard Options"=w194, "Gases Used"=w200, "Fraction of Inhaled Oxygen"=w202, "BallZero Options"=w196, "IRS Options"=w195) -> ("Resonator ID"=w198:string, "Sample Selected"=w199:string, "Sample Type"=w193:T9)  [unwired: 4 in, 1 out]
            }
            frame "QA-Start/End" {
              n46 = Unbundle By Name(w213) -> ("Sample Type"=w212:T9)
              n47 = Index Array(array=w216, index=0) -> (element=w214:string)
              n48 = case shown="\"BallZero\"" w212 {
                tunnel: [Sample_Type."BallZero" ("Sample Type") Sample_Type."Empty Resonator" ("Sample Type") Sample_Type."IRS" ("Sample Type")] -> w211
                tunnel: [FALSE ("s") TRUE ("s") FALSE ("s")] -> w205
                tunnel: w208 -> [_ _ w223]
                tunnel: [w217 string[] [] w223] -> w207
                tunnel: w206 -> [w217 _ _]
                frame "Empty Resonator", Default {
                  # "BallZero First then IRS"
                }
                frame "IRS" {
                  # "After IRS, end session"
                }
                frame "BallZero" {
                  # "After BallZero --> IRS"
                }
              }
              n49 = Index Array(array=w207, index=0) -> (element=w209:string)
              n50 = Not(x=w205) -> (.not. x?=w204:bool)
            }
            frame "QA-Mid" {
              n51 = Unbundle By Name(w228) -> ("Sample Type"=w229:T9)
              n52 = Index Array(array=w236, index=0) -> (element=w235:string)
              n53 = case shown="\"Empty Resonator\", Default" w229 {
                tunnel: [Sample_Type."IRS" ("Sample Type") Sample_Type."Empty Resonator" ("Sample Type")] -> w230
                tunnel: [FALSE ("s") TRUE ("s")] -> w227
                frame "Empty Resonator", Default {
                }
                frame "IRS" {
                }
              }
              n54 = Index Array(array=w232, index=0) -> (element=w231:string)
              n55 = Not(x=w227) -> (.not. x?=w226:bool)
            }
            frame "QA-Weekly" {
              n56 = Unbundle By Name(w243) -> ("Sample Type"=w244:T9)
              n57 = Index Array(array=w254, index=0) -> (element=w253:string)
              n58 = case shown="\"Empty Resonator\", Default" w244 {
                tunnel: [Sample_Type."BallZero" ("Sample Type") Sample_Type."Irradiated Tooth" ("Sample Type") Sample_Type."IRS" ("Sample Type") Sample_Type."Empty Resonator" ("Sample Type")] -> w251
                tunnel: [FALSE ("s") FALSE ("s") FALSE ("s") TRUE ("s")] -> w242
                tunnel: w250 -> [w255 _ _ _]
                tunnel: [w255 w258 w261 string[] []] -> w247
                tunnel: w246 -> [_ _ w261 _]
                tunnel: w245 -> [_ w258 _ _]
                frame "Empty Resonator", Default {
                  # "BallZero first"
                }
                frame "IRS" {
                  # "Tooth 3rd"
                }
                frame "BallZero" {
                  # "IRS Second"
                }
                frame "Irradiated Tooth" {
                  # "Exit after 30Gy tooth"
                }
              }
              n59 = Not(x=w242) -> (.not. x?=w241:bool)
              n60 = Index Array(array=w247, index=0) -> (element=w248:string)
            }
            frame "Check Calibration" {
              w267 = FALSE ("s")
              # "Prompting is handled within Check Cal Routine"
              n61 = Index Array(array=w274, index=0) -> (element=w273:string)
              n62 = Index Array(array=w268, index=0) -> (element=w269:string)
            }
          }
        }
        frame 1 {
          n63 = call "Initialize Vitro Session.vi"("Tooth Strings"=w283, "Tooth Data File"=w284, "resonator labels"=w285) -> ("Resonator ID"=w279:string, "Tooth ID"=w280:string)  [unwired: 1 in]
        }
        frame 2 {
          n64 = call "Initialize Vivo Session.vi"("resonator labels"=w299, "Measurement Information In"=w290, "Volunteer Selections"=w298, "In Vivo Data File"=w297, "Sample Selection"=w296, "Tooth Position"=w294) -> ("Measurement Information Out"=w289:T7, "Sample Selection"=w291:string, "Sample Type"=w287:T9, "Measurement Site"=w295:string, "Selected Volunteer ID"=w293:string, "Resonator ID"=w292:string)  [unwired: 3 in, 1 out]
        }
      }
      n65 = To Upper Case(1:w13) -> (0:w83:string)
      n66 = To Upper Case(1:w11) -> (0:w82:string)
      n67 = Bundle By Name(cluster=w32, "Non-standard session?"=w84, "QA Mode"=w48, "Resonator Operator"=w83, "Computer Operator"=w82, "Session Type"=w89, "Tooth/Sample ID"=w81, "Volunteer ID"=w88, "Resonator"=w87, "Measurement Site"=w86, "Gases Available"=w85, "Sample Type"=w40, "QA Session?"=w52, "Number of sites"=w30) -> (w54:T7)
      n68 = Unbundle By Name(w32) -> ("DAQ Mode"=w37:enum16{"Engineering", "Dosimetry", "Oximetry"})
      n69 = Unbundle By Name(w39) -> ("Sensitivity"=w35:u16)
      n70 = Equal?(x=w37, y=enum16{"Engineering", "Dosimetry", "Oximetry"}."Dosimetry" ("DAQ Mode")) -> (x = y?=w36:bool)
      n71 = Select(t=u16 17, s=w36, f=w35) -> (s? t:f=w33:u16)
      n72 = Equal?(x=Sample_Type."IRS" ("Sample Type"), y=w40) -> (x = y?=w41:bool)
      n73 = Select(t=u16 18 ("Sensitivity"), s=w41, f=w33) -> (s? t:f=w43:u16)
      n74 = Equal?(x=w48, y=T6."QA-Start/End" ("QA Mode")) -> (x = y?=w60:bool)
      n75 = Equal?(x=w48, y=T6."QA-Mid" ("QA Mode")) -> (x = y?=w59:bool)
      n76 = Equal?(x=w48, y=T6."QA-Weekly" ("QA Mode")) -> (x = y?=w58:bool)
      n77 = Bundle By Name(cluster=w39, "Sensitivity"=w43) -> (→"Hardware Parameters Out":T2)
      n78 = Compound Arithmetic op=OR(w60, w59, w58) -> (w57:bool)
      n79 = case shown="True" w57 {
        tunnel: [w300 cluster{"Enum":T5, "Data":variant}[] [{"Enum"=enum."Configure Hardware", "Data"=variant}, {"Enum"=enum."Initialize Set", "Data"=variant}, {"Enum"=enum."Pre-Scan", "Data"=variant}]] -> w79
        tunnel: w40 -> [_ w307]
        tunnel: w48 -> [w305 _]
        frame False {
          n80 = Equal?(x=T6."Check Calibration" ("QA Mode"), y=w305) -> (x = y?=w303:bool)
          n81 = Select(t=cluster{"Enum":T5, "Data":variant}[] [{"Enum"=enum."Check Calibration", "Data"=variant}, {"Enum"=enum."Configure Hardware", "Data"=variant}, {"Enum"=enum."Initialize Set", "Data"=variant}, {"Enum"=enum."Pre-Scan", "Data"=variant}], s=w303, f=cluster{"Enum":T5, "Data":variant}[] [{"Enum"=enum."Idle", "Data"=variant}]) -> (s? t:f=w300:cluster{"Enum":T5, "Data":variant}[])
        }
        frame True {
          # "Prompts"
          n82 = case shown="\"IRS\"" w307 {
            frame "Empty Resonator", Default {
            }
            frame "IRS" {
              n83 = One Button Dialog(message="Please place IRS sample in the magnet and press OK") -> ()  [unwired: 1 in, 1 out]
            }
            frame "BallZero" {
              n84 = One Button Dialog(message="Please place BallZero sample in the magnet and press OK") -> ()  [unwired: 1 in, 1 out]
            }
            frame "Irradiated Tooth" {
              n85 = One Button Dialog(message="Please place 30Gy tooth sample in the magnet and press OK") -> ()  [unwired: 1 in, 1 out]
            }
            frame "Non-irradiated Tooth" {
            }
          }
        }
      }
      n86 = case shown="False" w49 {
        tunnel: w54 -> [w102 w109]
        tunnel: [w100 w108] -> w53
        tunnel: w39 -> [w99 _]
        tunnel: [w98 _] -> w46
        frame False {
          n87 = Unbundle By Name(w102) -> ("Session Number"=w103:i32)
          n88 = Increment(x=w103) -> (x+1=w106:i32)
          n89 = Bundle By Name(cluster=w102, "Session Number"=w106, "Skip End Session Save"=FALSE) -> (w101:T7)
          n90 = call "Write Key I32.vi"("Value to write"=w106, "key"="session_number", "section"="logging") -> ("error out"=w96:errorcluster)  [unwired: 8 in]
          n91 = call "Create New Data Directory.vi"("Measurement Information In"=w101, "Hardware Parameters In"=w99) -> ("error out"=w95:errorcluster, "Measurement Information Out"=w100:T7)  [unwired: 8 in]
          n92 = Merge Errors(w96, w95) -> (w98:errorcluster)
        }
        frame True {
          n93 = Bundle By Name(cluster=w109, "Skip End Session Save"=TRUE) -> (w108:T7)
          n94 = One Button Dialog(message="You have completed the QA.") -> ()  [unwired: 1 in, 1 out]
        }
      }
      n95 = Select(t=cluster{"Enum":T5, "Data":variant}[] [{"Enum"=enum."End Session", "Data"=variant}], s=w49, f=w79) -> (s? t:f=w78:cluster{"Enum":T5, "Data":variant}[])
    }
    frame True {
      n96 = Bundle By Name(cluster=w312, "Skip End Session Save"=TRUE, "QA Session?"=FALSE, "Sample Type"=Sample_Type."Empty Resonator", "QA Mode"=T6."Select QA Mode") -> (w314:T7)
    }
  }
  "Measurement Information Out" <- w7
  "QSM Response" <- w10
  "Spectral Data Out" <- w6
  "error out" <- w5
  "Acquisition Parameters Out" <- w1
